vi "Initialize.vi"(8 "error in (no error)":errorcluster, 11 "Sensor & Control in":refnum<class "Control.lvclass">) -> (0 "error out":errorcluster, 3 "Sensor & Control out":refnum<class "Control.lvclass">)   [LabVIEW 2013, in "Control.lvib.lvlib" / "Control.lvclass"]
uses:
  Control.lvclass
  <vilib>/Instr/_visa.llb/VISA Configure Serial Port (Instr).vi
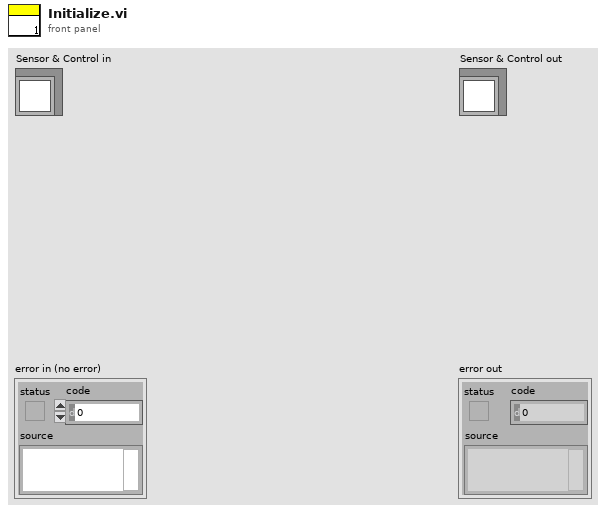
[diagram p1: front panel]
types:
  T1 = enum16{"open", "open or create", "create or replace", "create", "open (read-only)"}
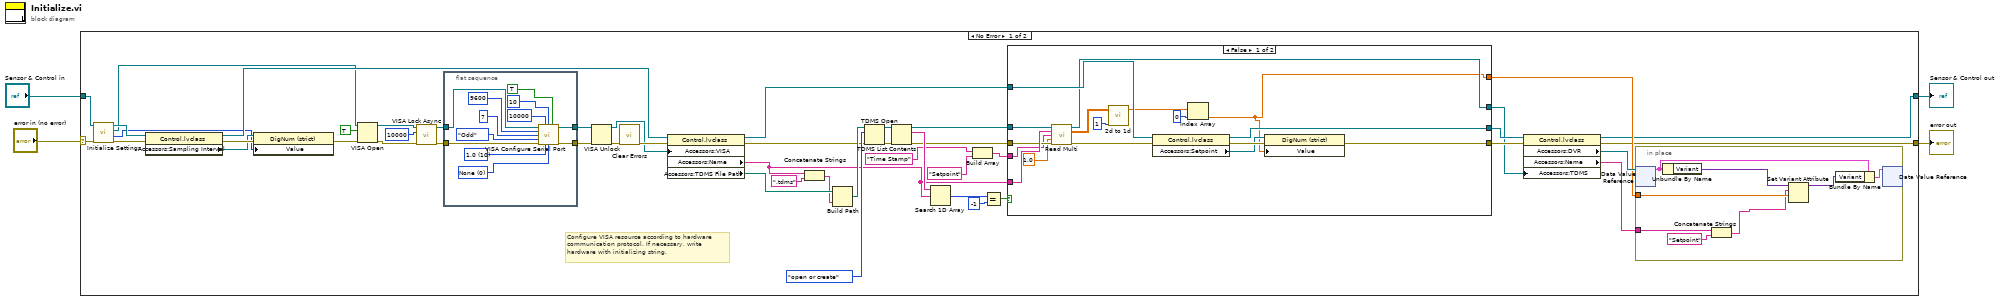
[diagram p0: block diagram]
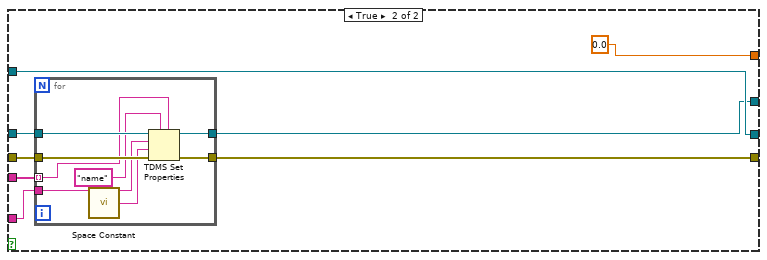
[diagram p2: hidden frame]
diagram:
  n1 = case shown="No Error" "error in (no error)" {
    selector: "error in (no error)" -> [w16 w107]
    tunnel: [w8 w107] -> w3
    tunnel: [w9 w106] -> w1
    tunnel: "Sensor & Control in" -> [w18 w106]
    frame No Error {
      # "Configure VISA resource according to hardware\ncommunication protocol. If necessary, write\nhardware with initializing string."
      n2 = call "Initialize Settings.vi"("error in (no error)"=w16, "Sensor & Control in"=w18) -> ("error out"=w11:errorcluster, "Sampling Interval 2"=w13:i32, "VISA out"=w15:refnum<visa-resource-name>, "Sensor & Control out"=w17:refnum<class "Control.lvclass">)  [unwired: 6 in]
      n3 = property class="Control.lvclass"(reference=w17, error in=w11) -> (reference out=w20:refnum<class "Control.lvclass">, error out=w19:errorcluster, "Accessors:Sampling Interval"=w14:refnum<vi>)
      n4 = property class="DigNum (strict)"(reference=w14, error in=w19, "Value"=w13) -> (error out=w12:errorcluster)  [unwired: 1 out]
      n5 = VISA Open(duplicate session (F)=TRUE, error in (no error)=w12, VISA resource name=w15) -> (VISA resource name=w26:refnum<visa-resource-name>, error out=w29:errorcluster)  [unwired: 2 in]
      n6 = call <vilib>:"VISA Lock Async.vi"("error in (no error)"=w29, "timeout (0)"=u32 10000, "VISA resource name"=w26) -> ("error out"=w28:errorcluster, "VISA resource name out"=w27:refnum<visa-resource-name>)  [unwired: 6 in, 1 out]
      n7 = flat-sequence {
        tunnel: w27 -> [w59]
        tunnel: w28 -> [w58]
        tunnel: [w57] -> w24
        tunnel: [w56] -> w23
        frame #0 {
          w55 = u16 0 items=["None", "XON/XOFF", "RTS/CTS", "XON/XOFF & RTS/CTS", "DTR/DSR", "XON/XOFF & DTR/DSR"] ("flow control (0:none)")
          w61 = u16 10 items=["1.0"=10, "1.5"=15, "2.0"=20] ("stop bits (10: 1 bit)")
          n8 = call-poly "VISA Configure Serial Port"("VISA resource name"=w59, "timeout (10sec)"=u32 10000, "termination char\n(0xA = '\\n' = LF)"=u8 10 ("termination char\n(0xA = '\\n' = LF)"), "Enable Termination\nChar (T)"=TRUE ("Enable Termination\nChar (T)"), "baud rate (9600)"=u32 9600, "data bits (8)"=u16 7, "parity (0:none)"=enum16{"None", "Odd", "Even", "Mark", "Space"}."Odd", "error in (no error)"=w58, "stop bits (10: 1 bit)"=w61, "flow control (0:none)"=w55) -> ("VISA resource name out"=w56:refnum<visa-resource-name>, "error out"=w57:errorcluster)  [unwired: 4 out]
        }
      }
      n9 = VISA Unlock(8:w24, 11:w23) -> (0:w33:errorcluster, 3:w32:refnum<visa-resource-name>)
      n10 = call <vilib>:"Clear Errors.vi"("error in (no error)"=w33) -> ("error out"=w43:errorcluster)  [unwired: 6 in]
      n11 = property class="Control.lvclass"(reference=w20, error in=w43, "Accessors:VISA"=w32) -> (reference out=w6:refnum<class "Control.lvclass">, error out=w5:errorcluster, "Accessors:Name"=w7:string, "Accessors:TDMS File Path"=w39:path)
      n12 = Concatenate Strings(w7, ".tdms" ("name or relative path")) -> (w21:string)
      n13 = Build Path(base path=w39, name or relative path=w21) -> (appended path=w42:path)
      n14 = TDMS Open(8:w5, 10:T1."open or create" ("operation (0:open)"), 11:w42) -> (0:w41:errorcluster, 3:w38:refnum<k34>)  [unwired: 4 in]
      n15 = TDMS List Contents(4:w41, 7:w38) -> (0:w47:errorcluster, 2:w50:string[], 3:w48:refnum<k34>)  [unwired: 1 in, 1 out]
      n16 = Search 1D Array(1D array=w50, element=w7) -> (index of element=w51:i32)  [unwired: 1 in]
      n17 = Build Array("Time Stamp" ("Channel"), "Setpoint" ("string")) -> (w46:string[])
      n18 = Equal?(x=w51, y=-1) -> (x = y?=w49:bool)
      n19 = case shown="False" w49 {
        tunnel: w48 -> [w84 w97]
        tunnel: [w73 w93] -> w36
        tunnel: w47 -> [w87 w95]
        tunnel: w7 -> [w88 w96]
        tunnel: w6 -> [w89 w92]
        tunnel: w46 -> [w76 w94]
        tunnel: [w83 w92] -> w35
        tunnel: [w75 w91] -> w31
        tunnel: [w74 0.0 ("Numeric Control")] -> w30
        frame False {
          n20 = call "Read Multi.vi"("tdms file in"=w84, "group"=w88, "Channel"=w76, "Numeric"=1.0, "error in (no error)"=w87) -> ("tdms file out"=w75:refnum<k34>, "Array"=w81:dbl[][], "error out"=w86:errorcluster)  [unwired: 7 in, 1 out]
          n21 = call "2d to 1d.vi"("index"=1, "array"=w81) -> ("output array"=w80:dbl[])  [unwired: 9 in]
          n22 = property class="Control.lvclass"(reference=w89, error in=w86) -> (reference out=w83:refnum<class "Control.lvclass">, error out=w79:errorcluster, "Accessors:Setpoint"=w78:refnum<vi>)
          n23 = Index Array(array=w80, index=0) -> (element=w74:dbl)
          n24 = property class="DigNum (strict)"(reference=w78, error in=w79, "Value"=w74) -> (error out=w73:errorcluster)  [unwired: 1 out]
        }
        frame True {
          n25 = for {
            tunnel: w95 -> [w105]
            tunnel: [w104] -> w93
            tunnel: w97 -> [w103]
            tunnel: w96 -> [w102]
            tunnel: w94 -> [w101] mode=indexing
            tunnel: [w98] -> w91
            n26 = call <vilib>:"Space Constant.vi"() -> ("String"=w99:string)
            n27 = TDMS Set Properties(5:w101, 7:"name" ("property names"), 8:w105, 9:w99, 10:w102, 11:w103) -> (0:w104:errorcluster, 3:w98:refnum<k34>)  [unwired: 2 out]
          }
        }
      }
      n28 = property class="Control.lvclass"(reference=w35, error in=w36, "Accessors:TDMS"=w31) -> (reference out=w9:refnum<class "Control.lvclass">, error out=w8:errorcluster, "Accessors:DVR"=w37:refnum<data-value>, "Accessors:Name"=w10:string)
      n29 = in-place {
        in-place-border: w30 -> [w68]
        in-place-border: w10 -> [w66]
        n30 = in-place-dvr #1(w37) -> (w69:cluster{"Array":string[], "Variant":variant})  [unwired: 1 out]
        n31 = Unbundle By Name(w69) -> ("Variant"=w71:variant)
        n32 = Concatenate Strings(w66, "Setpoint" ("string")) -> (w65:string)
        n33 = Set Variant Attribute(Variant=w71, name=w65, value=w68) -> (Variant out=w70:variant)  [unwired: 1 in, 2 out]
        n34 = Bundle By Name(cluster=w69, "Variant"=w70) -> (w72:cluster{"Array":string[], "Variant":variant})
        n35 = in-place-dvr #1(w72) -> ()  [unwired: 2 out]
      }
    }
    frame Error {
    }
  }
  "error out" <- w3
  "Sensor & Control out" <- w1
